vi "S7_Init_Adapter_TCP.vi"(8 "error in":errorcluster, 10 "Timeout":u32=5000, 11 "TCP Connection Ref":refnum<k5>) -> (0 "error out":errorcluster, 2 "Connected":bool, 3 "TCP Connection Ref Out":refnum<k5>)   [LabVIEW 2017, in "S7 TCP.lvlib"]
uses:
  S7 TCP.lvlib
panel:
  out "Attempts":i32
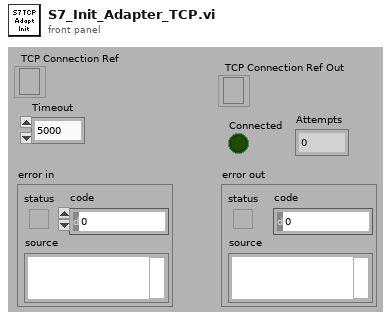
[diagram p1: front panel]
types:
  T1 = enum16{"Standard", "Buffered", "CRLF", "Immediate"}
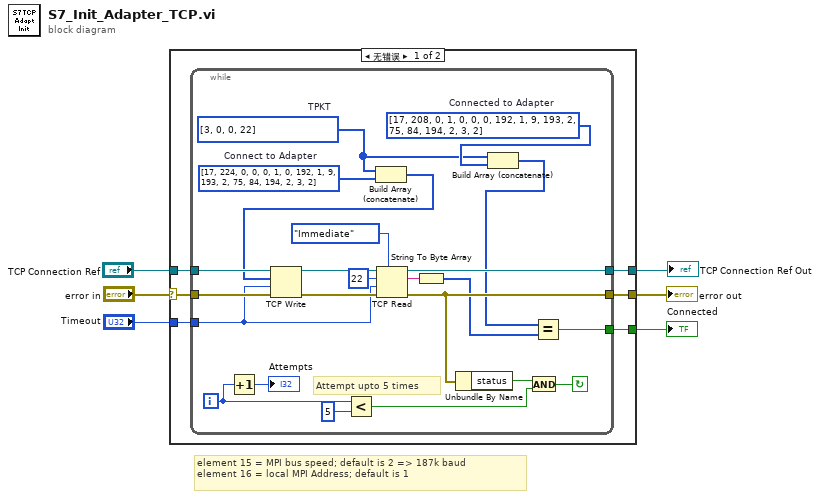
[diagram p0: block diagram]
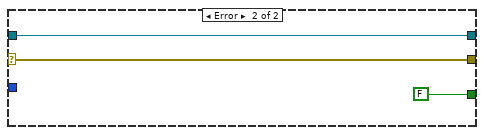
[diagram p2: hidden frame]
diagram:
  # "element 15 = MPI bus speed; default is 2 => 187k baud\nelement 16 = local MPI Address; default is 1"
  n1 = case shown="无错误" "error in" {
    selector: "error in" -> [w11 w38]
    tunnel: [w10 w37] -> w1
    tunnel: [w9 w38] -> w5
    tunnel: "TCP Connection Ref" -> [w12 w37]
    tunnel: [w8 FALSE] -> w4
    tunnel: "Timeout" -> [w7 _]
    frame No Error {
      n2 = while {
        tunnel: w12 -> [w28]
        tunnel: w11 -> [w27]
        tunnel: [w23] -> w10
        tunnel: [w24] -> w9
        tunnel: [w35] -> w8
        tunnel: w7 -> [w21]
        i -> [w33]
        stop <- w34 continue-if-true
        w16 = u8[] [17, 208, 0, 1, 0, 0, 0, 192, 1, 9, 193, 2, 75, 84, 194, 2, 3, 2]  # Connected to Adapter
        w15 = u8[] [3, 0, 0, 22]  # TPKT
        w18 = u8[] [17, 224, 0, 0, 0, 1, 0, 192, 1, 9, 193, 2, 75, 84, 194, 2, 3, 2]  # Connect to Adapter
        # "Attempt upto 5 times"
        n3 = Increment(x=w33) -> (x+1=→"Attempts":i32)
        n4 = Less?(x=w33, y=5) -> (x < y?=w31:bool)
        n5 = Build Array (concatenate)(w15, w18) -> (w17:u8[])
        n6 = TCP Write(connection ID=w28, data in=w17, error in (no error)=w27, 9:w21) -> (connection ID out=w26:refnum<k5>, error out=w25:errorcluster)  [unwired: 1 out]
        n7 = TCP Read(connection ID=w26, bytes to read=22, error in (no error)=w25, 7:T1."Immediate" ("mode (standard)"), 9:w21) -> (connection ID out=w23:refnum<k5>, data out=w19:string, error out=w24:errorcluster)
        n8 = String To Byte Array(string=w19) -> (unsigned byte array=w14:u8[])
        n9 = Unbundle By Name(w24) -> ("status"=w29:bool)
        n10 = Build Array (concatenate)(w15, w16) -> (w13:u8[])
        n11 = And(x=w29, y=w31) -> (x .and. y?=w34:bool)
        n12 = Equal?(x=w13, y=w14) -> (x = y?=w35:bool)
      }
    }
    frame Error {
    }
  }
  "error out" <- w5
  "Connected" <- w4
  "TCP Connection Ref Out" <- w1
